vi "niRFUtil WFM Interpolate Waveform (real wfm).vi"(0 "Waveform In":T1 {"y" min=0 max=127 format="%.2f"; "dx" format="%^.2e"; "x0" format="%^.2e"}, 5 "Rate (1)":i32=1, 7 "Offset (0)":i32) -> (4 "Waveform Out":T1 {"y" min=0 max=127 format="%.2f"; "dx" format="%^.2e"; "x0" format="%^.2e"})   [LabVIEW 2015, in "niRFUtil.lvlib"]
doc: "(c) Copyright 2006, National Instruments, Inc. This VI may not be duplicated, sold, or distributed without written consent from National Instruments."
uses:
  niRFUtil.lvlib
  Includes/niRFUtil INC Real Waveform.ctl
  Includes/niRFUtil INC Real Array.ctl
  <vilib>/Analysis/2dsp.llb/Upsample (DBL).vi
  <vilib>/Analysis/NI_AALPro.lvlib
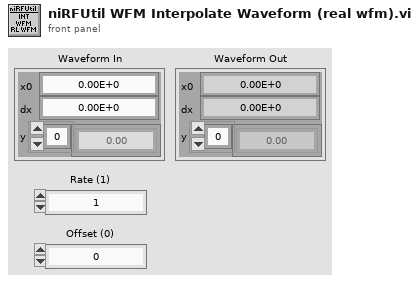
[diagram p1: front panel]
types:
  T1 = typedef "niRFUtil.lvlib/niRFUtil INC Real Waveform.ctl" = cluster{"x0":dbl, "dx":dbl, "y":T2}
  T2 = typedef "niRFUtil.lvlib/niRFUtil INC Real Array.ctl" = sgl[]
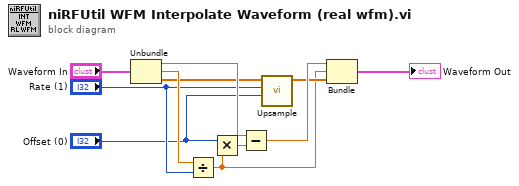
[diagram p0: block diagram]
diagram:
  n1 = Unbundle("Waveform In") -> ("x0"=w8:dbl, "dx"=w10:dbl, "y"=w6:T2)
  n2 = Divide(x=w10, y="Rate (1)") -> (x/y=w2:dbl)
  n3 = Multiply(x="Offset (0)", y=w2) -> (x*y=w9:dbl)
  n4 = Subtract(x=w8, y=w9) -> (x-y=w7:dbl)
  n5 = call-poly <vilib>:"Upsample.vi"("leading zeros"="Offset (0)", "upsampling factor"="Rate (1)", "X"=w6) -> ("Upsampled Array"=w4:dbl[])  [unwired: 8 out]
  n6 = Bundle(w7, w2, "Upsampled Array"=w4) -> (→"Waveform Out":cluster{dbl, dbl, "Upsampled Array":dbl[]})  [unwired: 1 out]
